vi "FindStartWord.vi"(5 "Index":i32, 6 "Data Buffer":u8[](array[numeric]) format="%.0x") -> (2 "Found":bool)   [LabVIEW 2010]
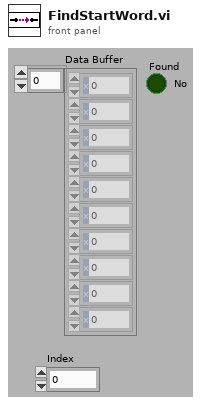
[diagram p1: front panel]
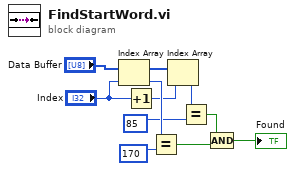
[diagram p0: block diagram]
diagram:
  n1 = Index Array(array="Data Buffer", index="Index") -> (element=w8:u8)
  n2 = Increment(x="Index") -> (x+1=w1:i32)
  n3 = Equal?(x=w8, y=u8 170) -> (x = y?=w5:bool)
  n4 = Index Array(array="Data Buffer", index=w1) -> (element=w9:u8)
  n5 = Equal?(x=w9, y=u8 85) -> (x = y?=w4:bool)
  n6 = Compound Arithmetic op=AND(w4, w5) -> (→"Found":bool)
